vi "Type Info.vi"(11 "ZIP Item in":refnum<class "ZIP Item.lvclass">) -> (1 "Description":string, 2 "Pretty Name":string, 3 "Type":string)   [LabVIEW 2019, in "ZIP.lvlib" / "ZIP Item.lvclass"]
doc: "Returns Type information about the solution item.\n----\nCopyright: MGI 2017\nAuthor: Derek Trepanier"
uses:
  ZIP Item.lvclass
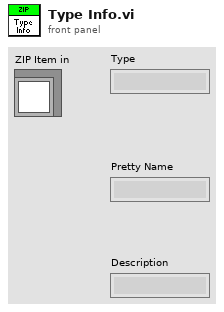
[diagram p1: front panel]
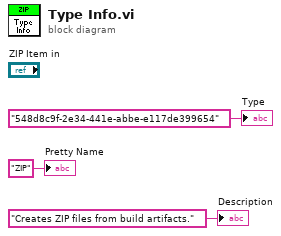
[diagram p0: block diagram]
diagram:
  "Pretty Name" <- "ZIP" ("Pretty Name")
  "Description" <- "Creates ZIP files from build artifacts." ("Description")
  "Type" <- "548d8c9f-2e34-441e-abbe-e117de399654" ("Type")
